vi "Write Encoder Type.vi"(0 "class data in":refnum<class "MB_ENGINE.lvclass">, 5 "U16":u16, 11 "error in (no error)":errorcluster) -> (4 "class data out":refnum<class "MB_ENGINE.lvclass">, 15 "error out":errorcluster)   [LabVIEW 2019, in "MB_ENGINE.lvclass"]
uses:
  MB_ENGINE.lvclass
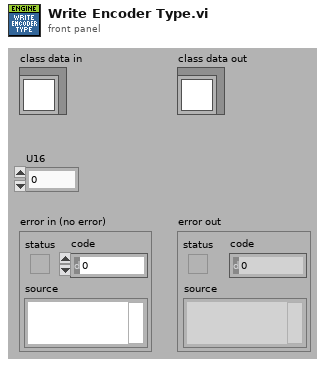
[diagram p1: front panel]
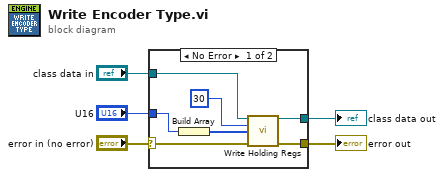
[diagram p0: block diagram]
diagram:
  n1 = case shown="No Error" "error in (no error)" {
    selector: "error in (no error)" -> [w11 w14]
    tunnel: [w10 w14] -> w4
    tunnel: "class data in" -> [w12 w13]
    tunnel: [w6 w13] -> w2
    tunnel: "U16" -> [w7 _]
    frame No Error {
      n2 = Build Array(w7) -> (w9:u16[])
      n3 = call-dynamic "Write Holding Regs.vi"("reference in"=w12, "starting address"=u16 30, "Regs"=w9, "error in (no error)"=w11) -> ("reference out"=w6:refnum<class "MB_ENGINE.lvclass">, "error out"=w10:errorcluster)  [unwired: 10 in]
    }
    frame Error {
    }
  }
  "error out" <- w4
  "class data out" <- w2
